vi "Nernst____Newtest.vi"() -> ()   [LabVIEW 2020]
panel:
  out "Temperature Status":i32(ring) items=["TemperatureUnknown"=0, "Stable"=1, "Tracking"=2, "Near"=5, "Chasing"=6, "Filling"=7, "Standby"=10, "Disabled"=13, "ImpedanceNotFunction"=14, "TempFailure"=15]
  out "Field Status":i32(ring) items=["MagnetUnknown"=0, "StablePersistent"=1, "WarmingSwitch"=2, "CoolingSwitch"=3, "StableDriven"=4, "Iterating"=5, "Charging"=6, "Discharging"=7, "CurrentError"=8, "MagnetFailure"=15]
  in  "Field":dbl[](array[numeric])
  out "Temp(A)":dbl
  out "Numeric":dbl
  in  "START":bool
  in  "T cold(A)":dbl
  in  "T hot(B)":dbl
  in  "Remote":bool=TRUE
  in  "IP address":string="10.128.163.210"
  in  "PPMS T(K)":dbl
  in  "Magnetic Field(Oe)":dbl
  in  "Pressure(GPa)":string
  in  "Heater Rate":string="50"
  in  "Heater Output":string="1"
  in  "Heater Mode":string="1"
  in  "Heater range":string="2"
  in  "Starting B":dbl
  in  "starting A":dbl
  out "save file Path":path=path "C:/DATA/Rui/testN1.dat.dat"
  in  "save file input":path=path "C:/DATA/Rui/testN1.dat"
  in  "Voltmeter":string="07"
  in  "T controller":string="12"
  out "Field\nStatus 2":i32(ring) items=["MagnetUnknown"=0, "StablePersistent"=1, "WarmingSwitch"=2, "CoolingSwitch"=3, "StableDriven"=4, "Iterating"=5, "Charging"=6, "Discharging"=7, "CurrentError"=8, "MagnetFailure"=15]
  in  "Cooling/Warming field":dbl[](array[numeric])
  in  "Field (Oe)":dbl[](array[numeric])=[0.0, 0.0, 0.0, 0.0, 0.0, 0.0, 0.0, 0.0]
  in  "Field Rate(Oe/sec)":dbl=100.0
  in  "Wait for T(s)":dbl=50.0
  in  "Wait for Field(s)":dbl=60.0
  in  "Wait For Temperature":bool=TRUE
  in  "T rate(K/min)":dbl=10.0
  in  "Delta T (TA-PPMST)":dbl[](array[numeric])=[0.0]
  in  "PPMST (K)":dbl[](array[numeric])=[0.0, 0.0]
  out "TIming(ms)":dbl
  in  "Time(ms)":dbl[](array[numeric])
  out "T gradient(K)":dbl
  in  "T gradient(K)":dbl[](array[numeric])
  out "Delta V(mV)":dbl
  out "T(A)(K)":dbl
  out "T(B)(K)":dbl
  in  "Tab Control":enum32{"V vs T", "V vs H"}(tab)
  out "XY Graph":cluster{"Y":dbl[], "Y":dbl[]}[](graph)
  out "XY Graph 2":cluster{"Y":dbl[], "Y":dbl[]}[](graph)
  in  "T Hot(A)":dbl[](array[numeric])
  in  "Delt V":dbl[](array[numeric])
  in  "T cold(B)":dbl[](array[numeric])
  # "Heater setups"
  # "GPIB Address"
  # "Save File Path"
  # "Environment setup"
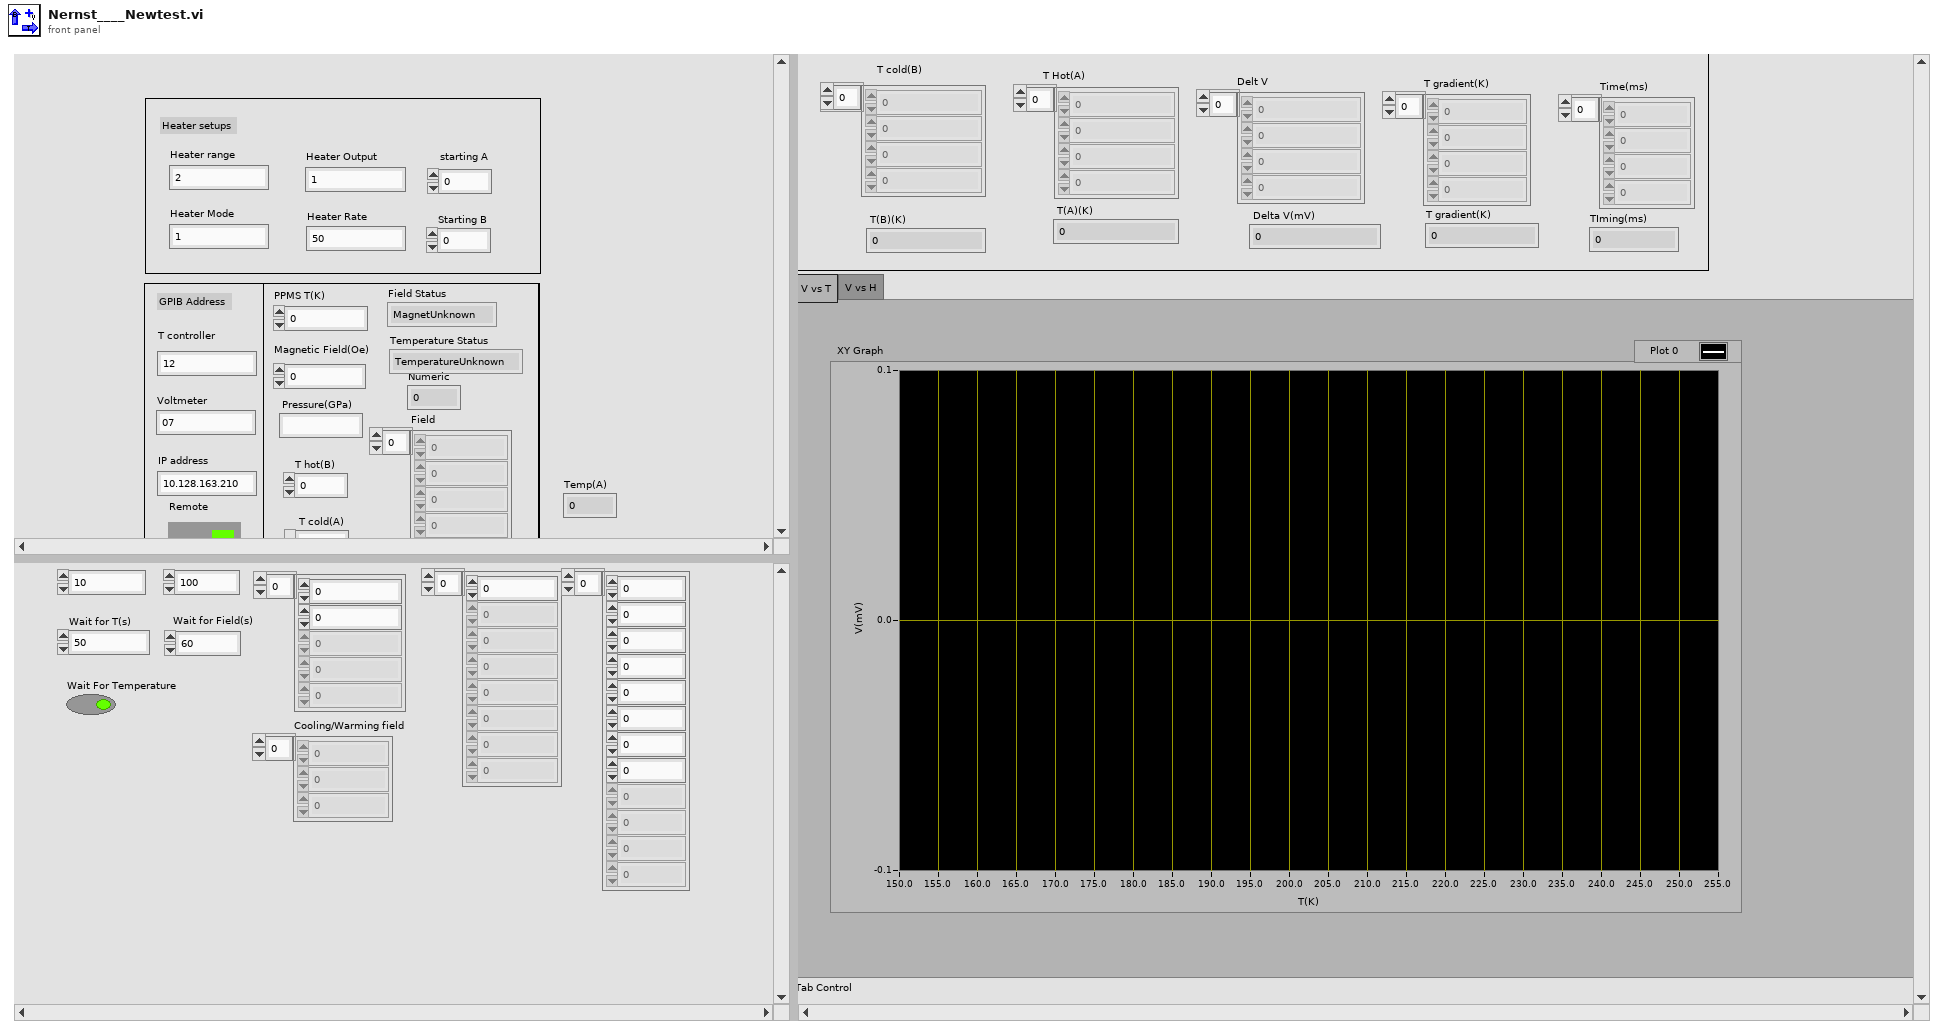
[diagram p1: front panel]
types:
  T1 = enum16{"open", "replace", "create", "open or create", "replace or create", "replace or create with confirmation"}
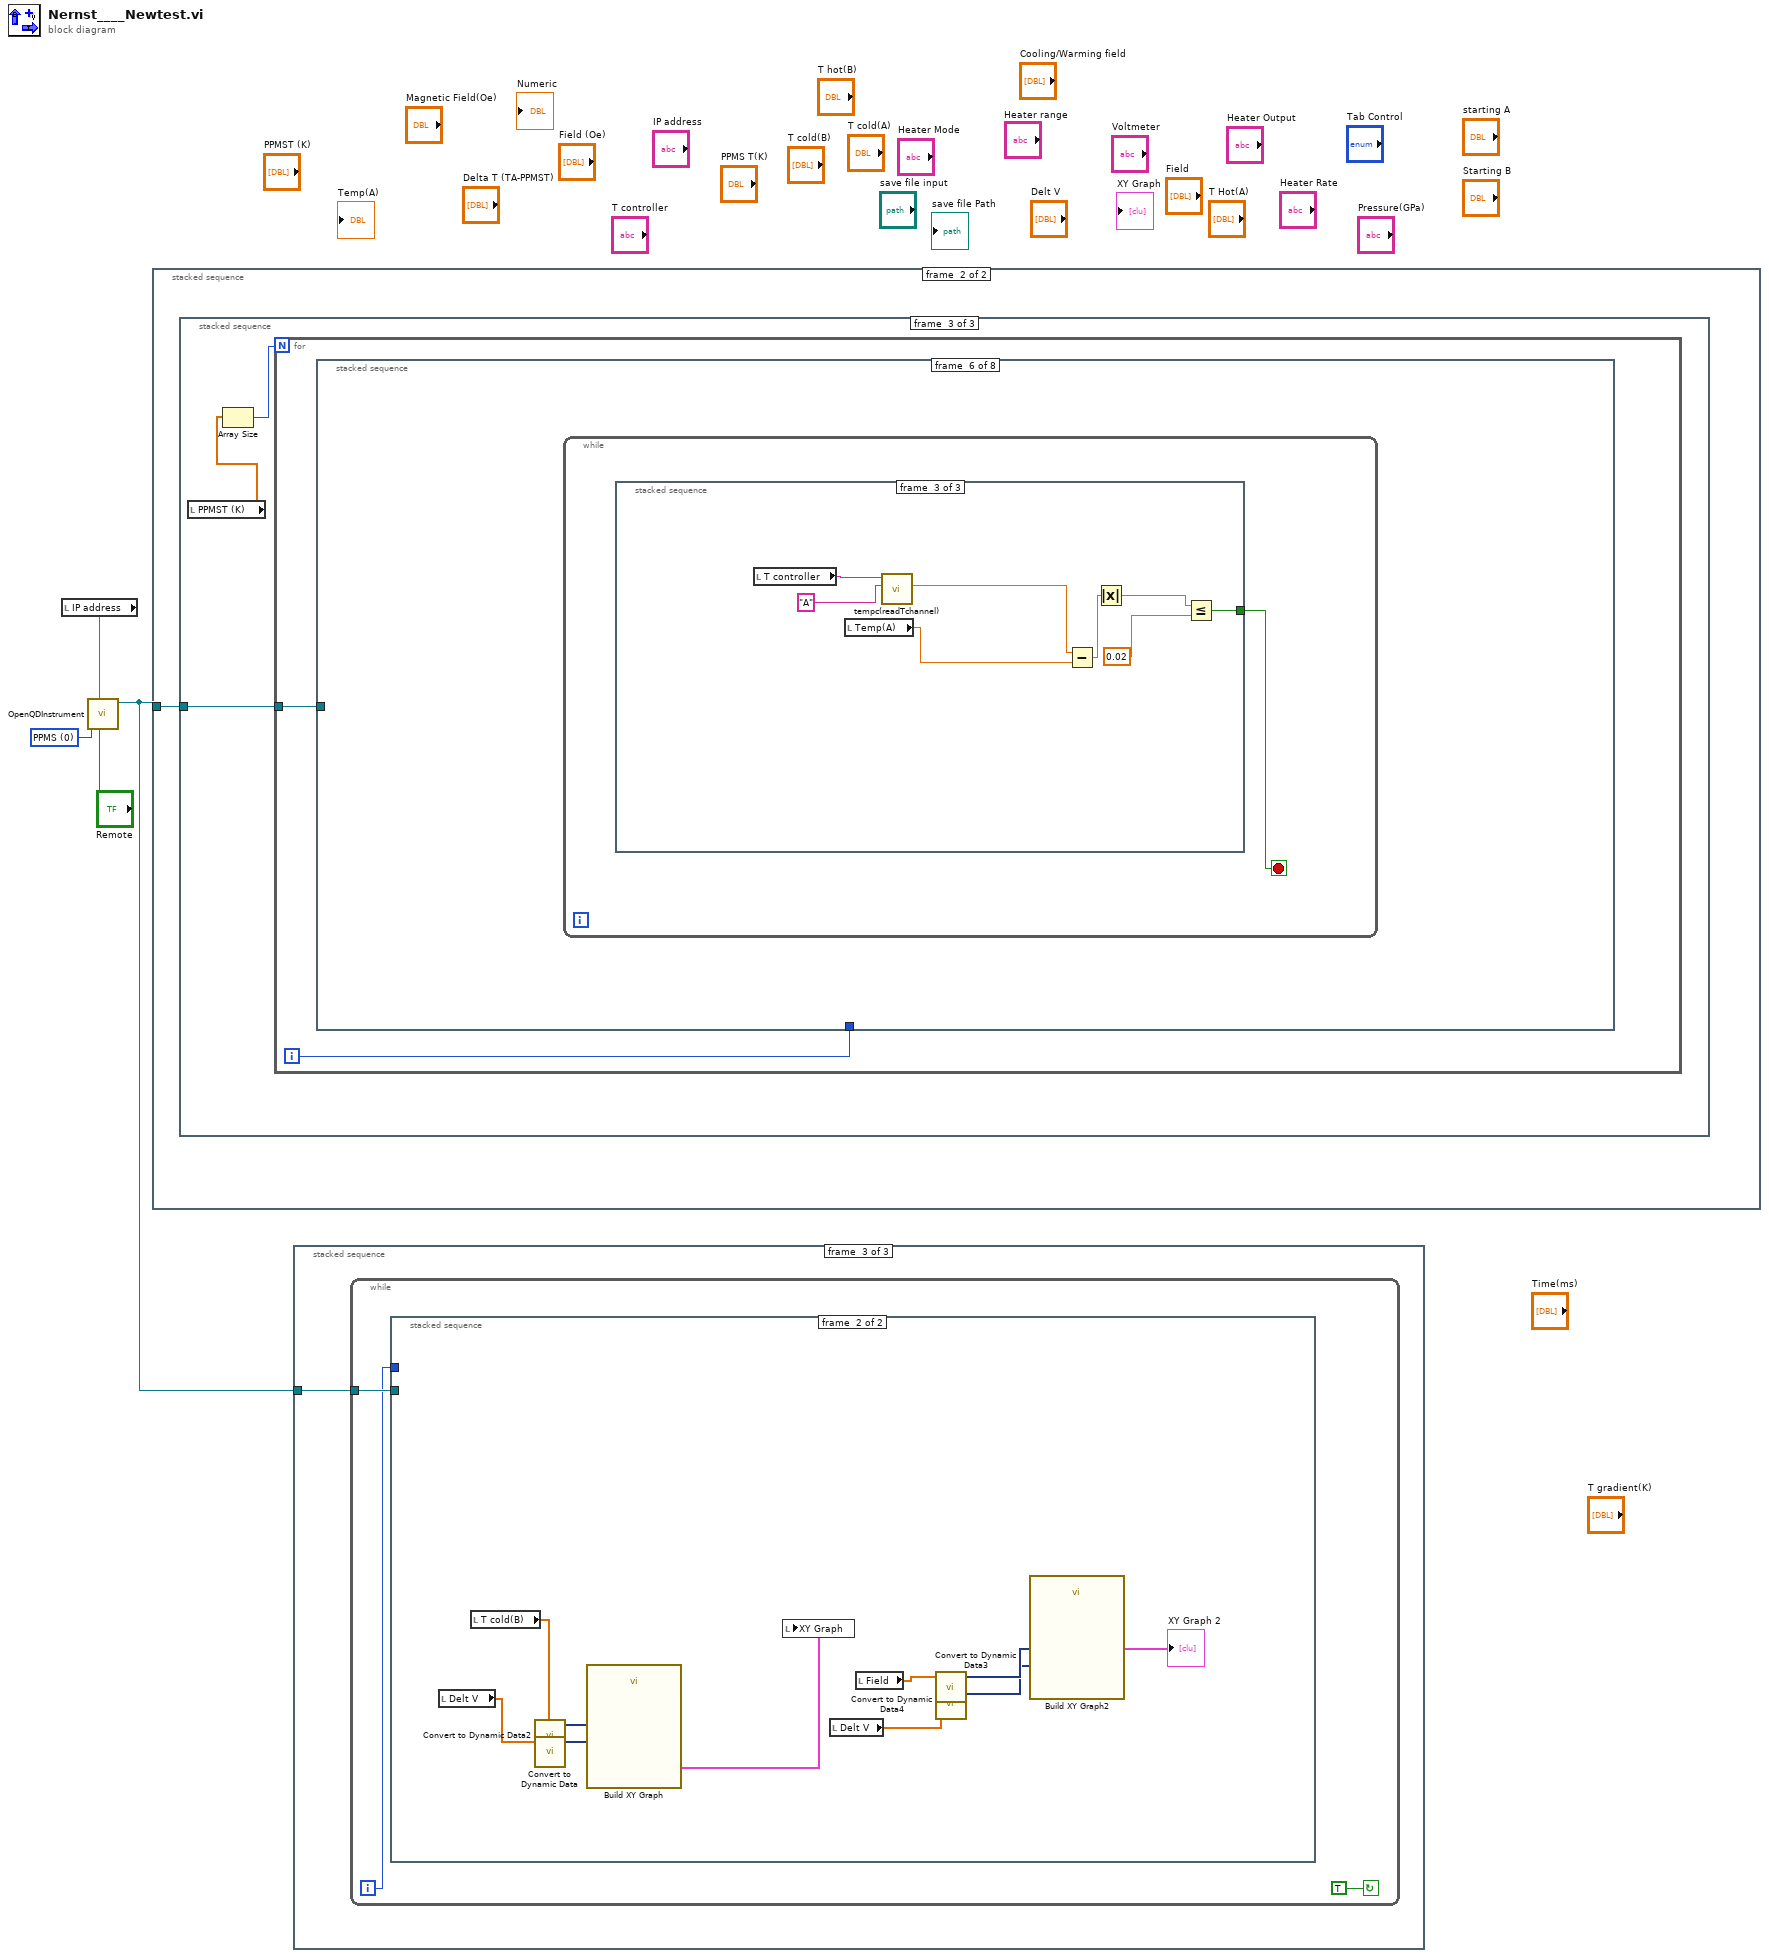
[diagram p0: block diagram]
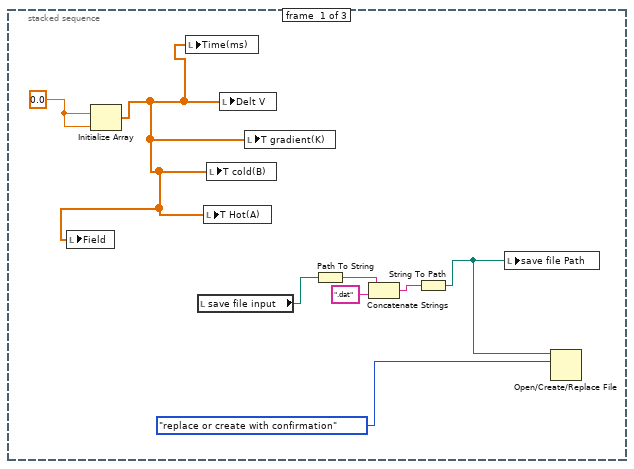
[diagram p2: hidden frame]
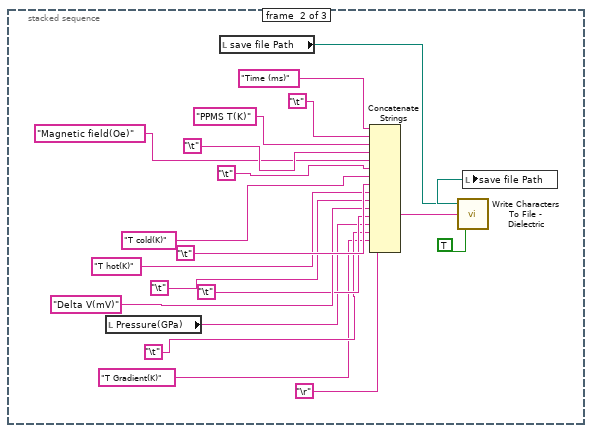
[diagram p3: hidden frame]
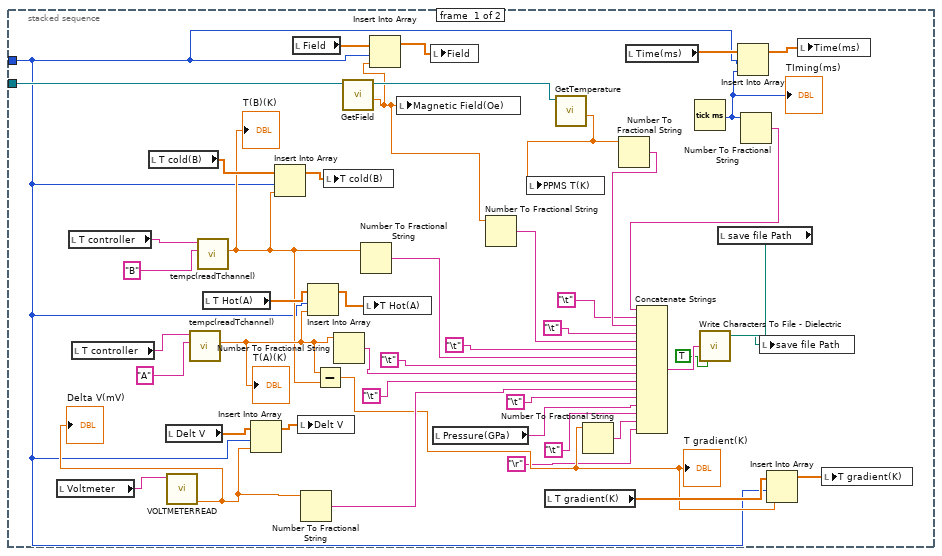
[diagram p4: hidden frame]
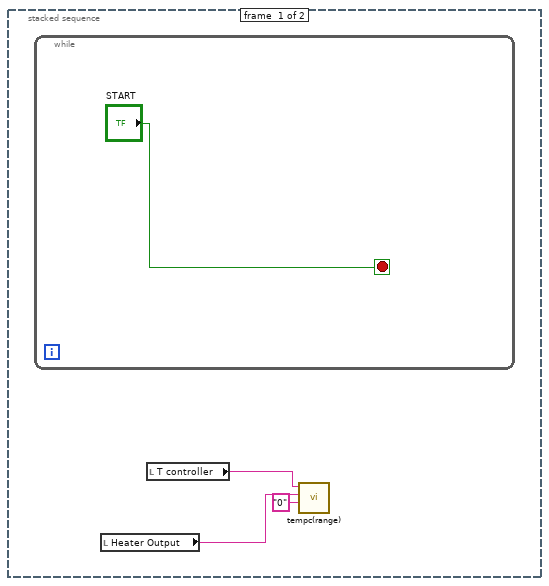
[diagram p5: hidden frame]
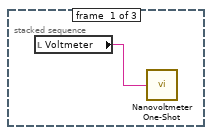
[diagram p6: hidden frame]
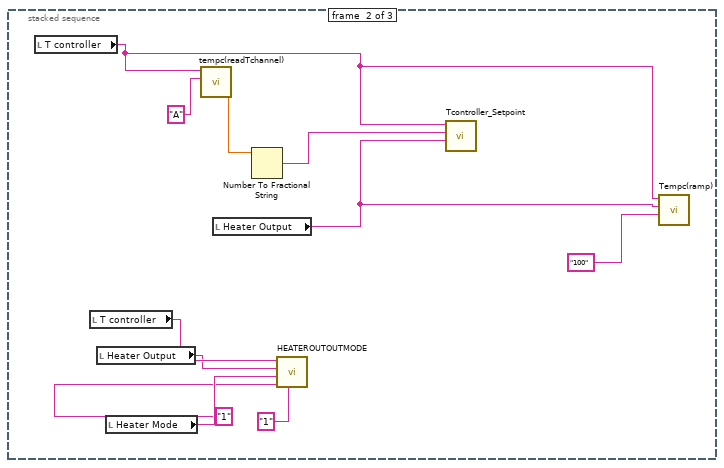
[diagram p7: hidden frame]
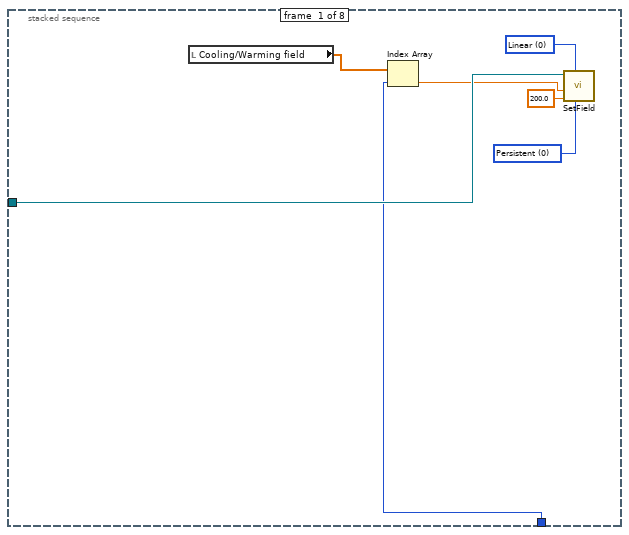
[diagram p8: hidden frame]
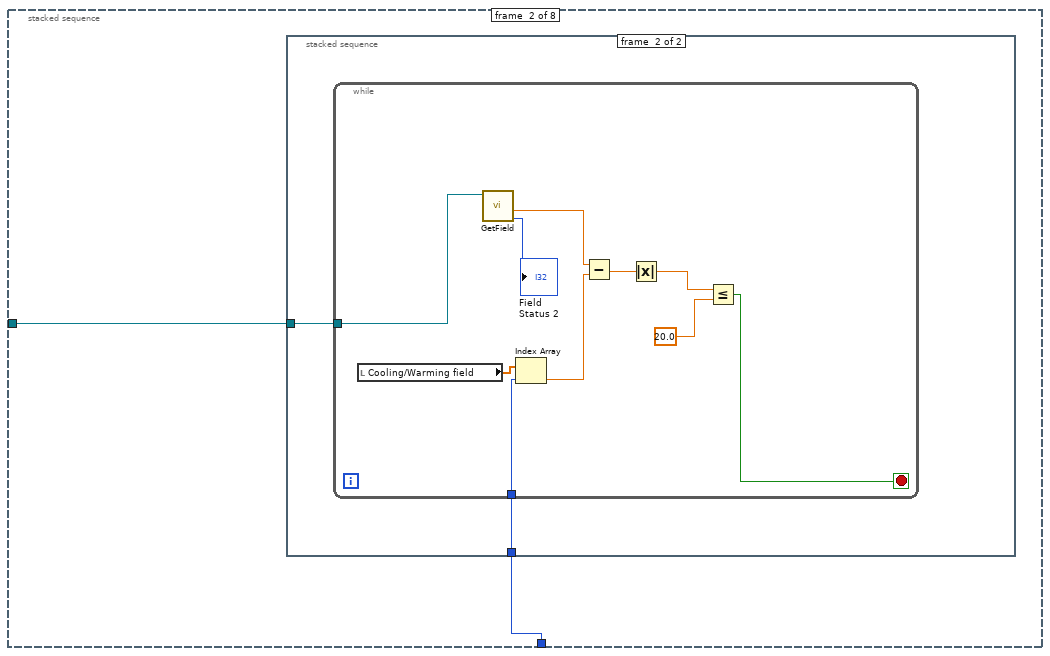
[diagram p9: hidden frame]
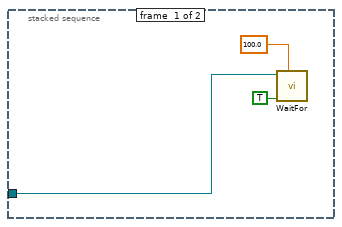
[diagram p10: hidden frame]
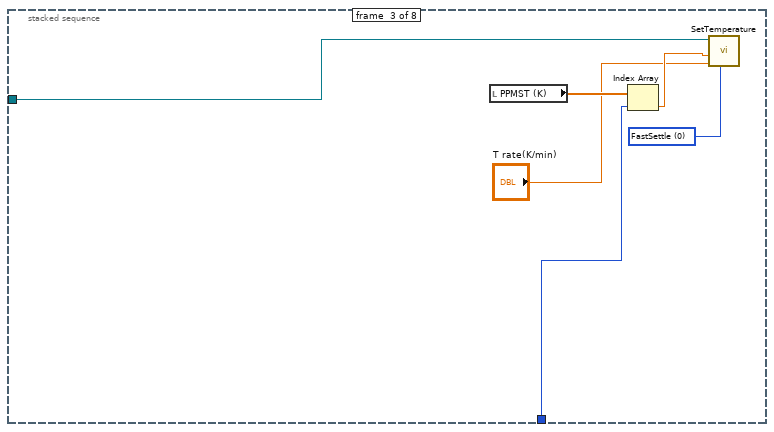
[diagram p11: hidden frame]
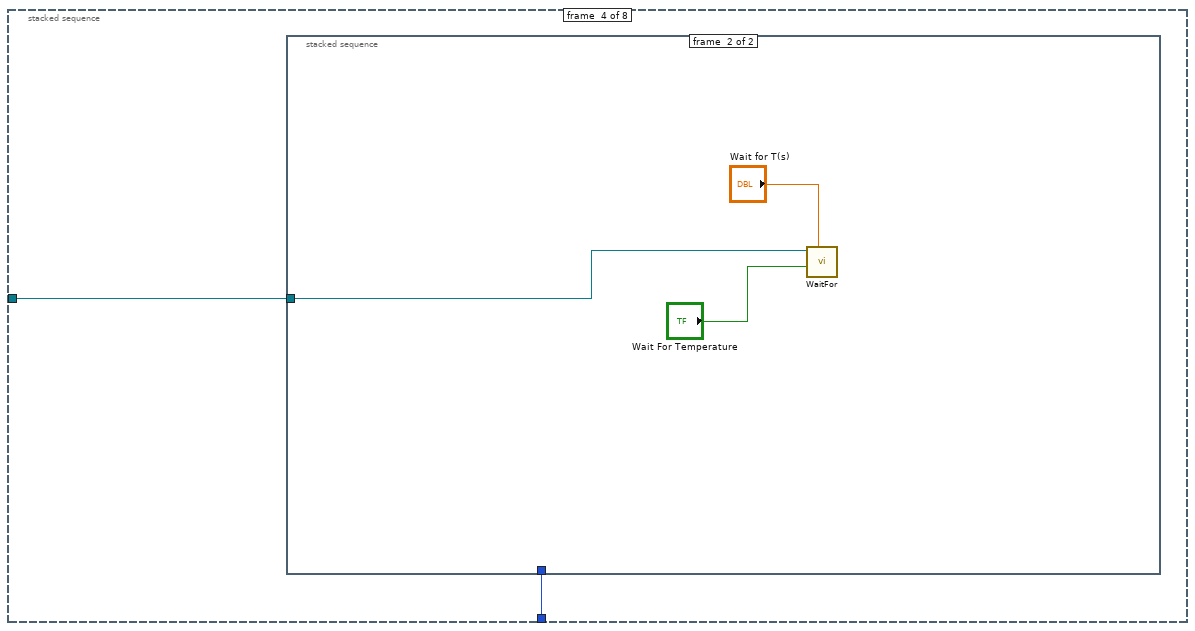
[diagram p12: hidden frame]
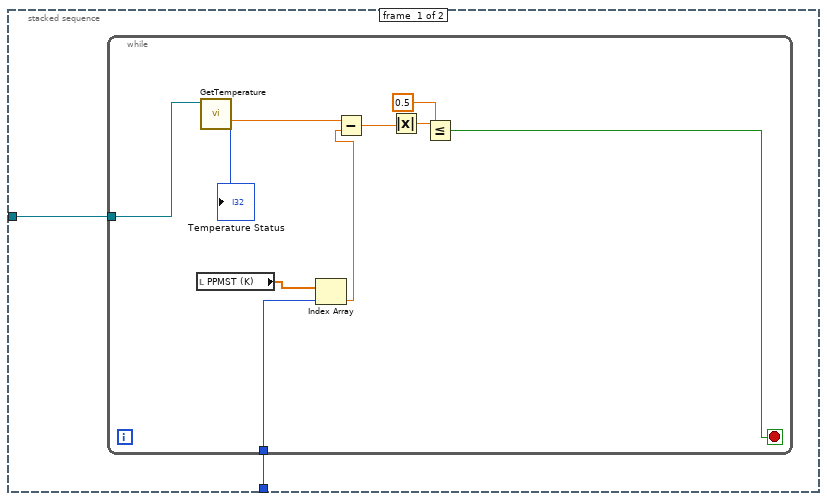
[diagram p13: hidden frame]
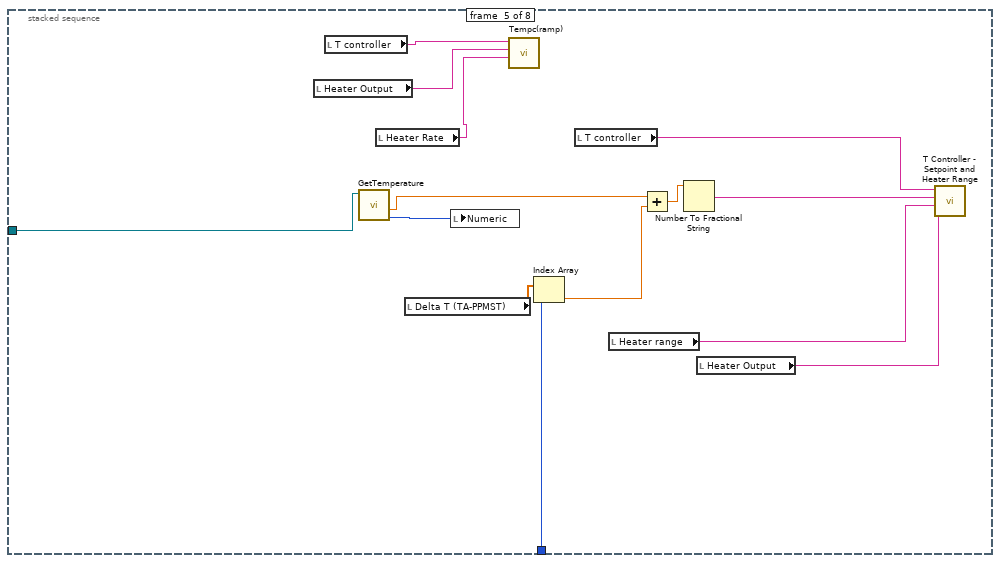
[diagram p14: hidden frame]
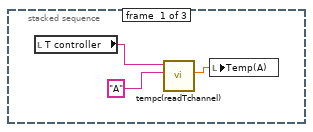
[diagram p15: hidden frame]
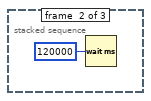
[diagram p16: hidden frame]
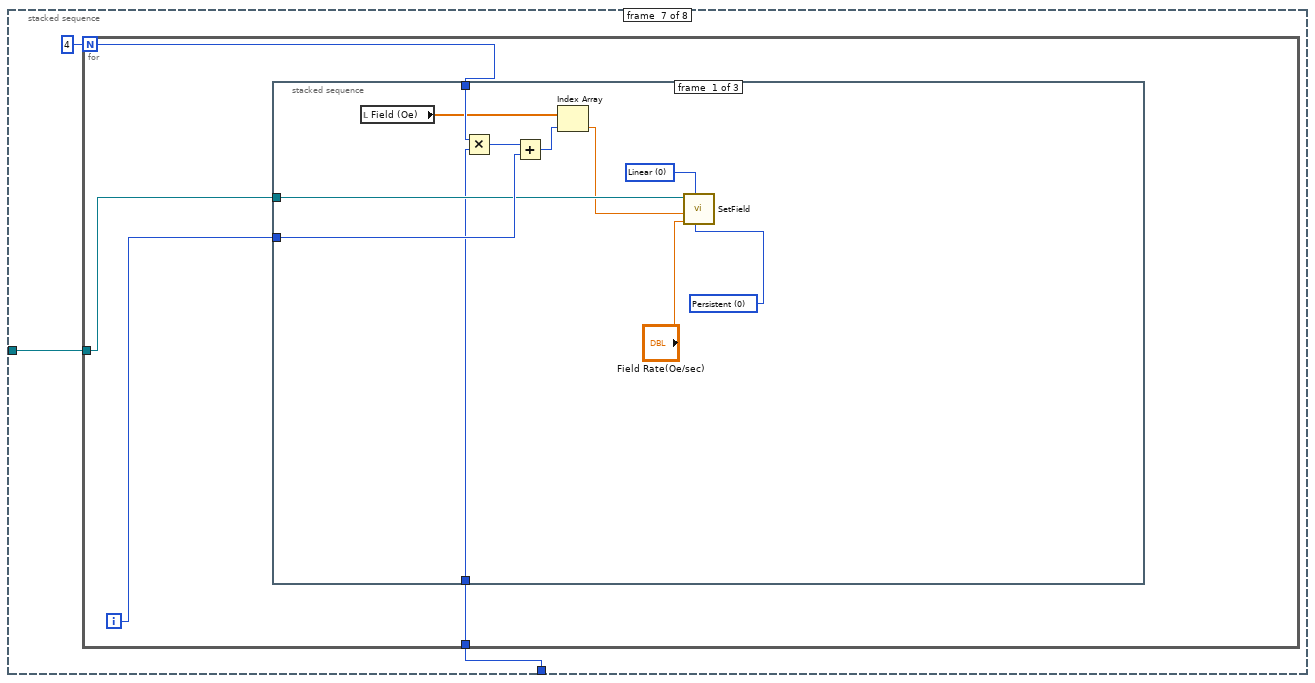
[diagram p17: hidden frame]
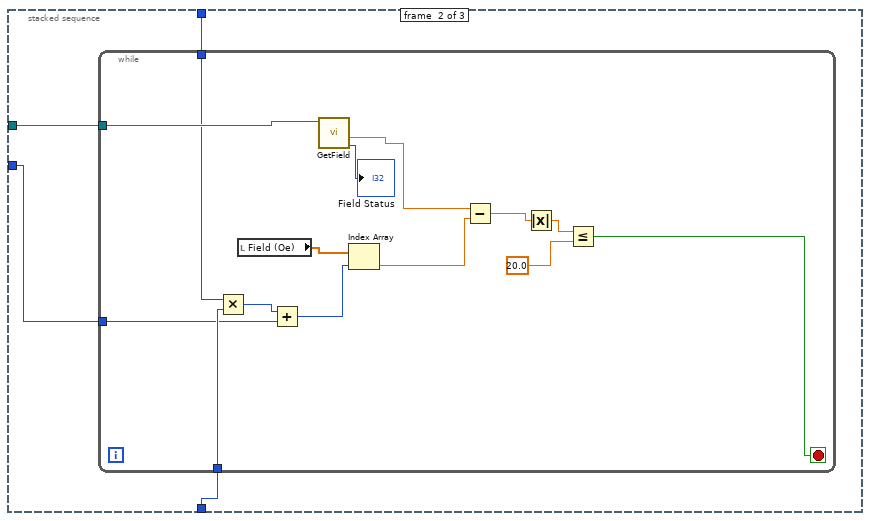
[diagram p18: hidden frame]
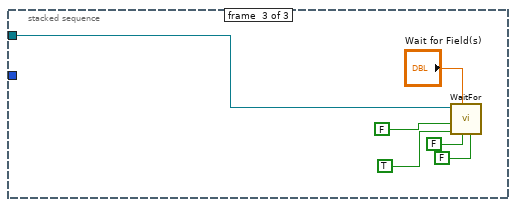
[diagram p19: hidden frame]
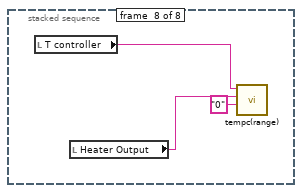
[diagram p20: hidden frame]
diagram:
  w2 = 0 items=["PPMS", "VersaLab", "DynaCool", "SVSM"] ("Instrument Type")
  n1 = local read "IP address"() -> (w4:string)
  n2 = call "OpenQDInstrument.vi"("Remote"="Remote", "IP Address"=w4, "Instrument Type"=w2) -> ("Instrument Ref"=w1:refnum<k24>)  [unwired: 5 in, 1 out]
  n3 = stacked-sequence {
    tunnel: w1 -> [_ w9]
    frame #0 {
      n4 = while {
        stop <- "START" stop-if-true
      }
      n5 = local read "Heater Output"() -> (w6:string)
      n6 = local read "T controller"() -> (w7:string)
      n7 = call "tempc(range).vi"("Heater ramge"="0", "Heater Output"=w6, "GPIB"=w7) -> ()  [unwired: 9 in]
    }
    frame #1 {
      n8 = stacked-sequence {
        tunnel: w9 -> [_ _ w24]
        frame #0 {
          n9 = local read "Voltmeter"() -> (w10:string)
          n10 = call "Nanovoltmeter One-Shot.vi"("GPIB address"=w10) -> ()
        }
        frame #1 {
          n11 = local read "T controller"() -> (w13:string)
          n12 = local read "T controller"() -> (w18:string)
          n13 = local read "Heater Output"() -> (w17:string)
          n14 = local read "Heater Mode"() -> (w16:string)
          n15 = call "tempc(readTchannel).vi"("input"="A", "address string"=w13) -> ("Temp"=w20:dbl)  [unwired: 9 in]
          n16 = local read "Heater Output"() -> (w12:string)
          n17 = Number To Fractional String(number=w20) -> (F-format string=w19:string)  [unwired: 3 in]
          n18 = call "HEATEROUTOUTMODE.vi"("poweruo enable"="1", "Input"="1", "Mode"=w16, "OUtput"=w17, "GPIB"=w18) -> ()  [unwired: 7 in]
          n19 = call "Tcontroller_Setpoint.vi"("OUTPUT"=w12, "SETPOINT"=w19, "GPIB"=w13) -> ()  [unwired: 9 in]
          n20 = call "Tempc(ramp).vi"("Rate Value"="100", "Output"=w12, "DPIB Add"=w13) -> ()  [unwired: 9 in]
        }
        frame #2 {
          n21 = local read "PPMST (K)"() -> (w23:dbl[])
          n22 = Array Size(array=w23) -> (size(s)=w22:i32)
          n23 = for {
            N: w22 -> [_]
            tunnel: w24 -> [w26]
            i -> [w25]
            n24 = stacked-sequence {
              tunnel: w26 -> [w33 w35 w56 w58 w79 _ w103 _]
              tunnel: w25 -> [w31 w34 w51 w57 w74 _ w101 _]
              frame #0 {
                w27 = 0 items=["Persistent", "Driven"] ("Mode")
                w28 = 0 items=["Linear", "NoOvershoot", "Oscillate"] ("Approach")
                n25 = local read "Cooling/Warming field"() -> (w32:dbl[])
                n26 = Index Array(array=w32, index=w31) -> (element=w30:dbl)
                n27 = call "SetField.vi"("Mode"=w27, "Approach"=w28, "Rate"=200.0, "Field"=w30, "Instrument Ref In"=w33) -> ()  [unwired: 2 in, 3 out]
              }
              frame #1 {
                n28 = stacked-sequence {
                  tunnel: w35 -> [w38 w40]
                  tunnel: w34 -> [_ w39]
                  frame #0 {
                    n29 = call "WaitFor.vi"("Delay"=100.0, "Wait For Field"=TRUE, "Instrument Ref In"=w38) -> ()  [unwired: 7 in, 2 out]
                  }
                  frame #1 {
                    n30 = while {
                      tunnel: w40 -> [w50]
                      tunnel: w39 -> [w48]
                      stop <- w41 stop-if-true
                      n31 = local read "Cooling/Warming field"() -> (w49:dbl[])
                      n32 = call "GetField.vi"("Instrument Ref In"=w50) -> ("Field\nStatus"=→"Field\nStatus 2":i32, "Field"=w47:dbl)  [unwired: 4 in, 3 out]
                      n33 = Index Array(array=w49, index=w48) -> (element=w46:dbl)
                      n34 = Subtract(x=w47, y=w46) -> (x-y=w44:dbl)
                      n35 = Absolute Value(x=w44) -> (abs(x)=w43:dbl)
                      n36 = Less Or Equal?(x=w43, y=20.0) -> (x <= y?=w41:bool)
                    }
                  }
                }
              }
              frame #2 {
                w52 = 0 items=["FastSettle", "NoOvershoot"] ("Approach")
                n37 = local read "PPMST (K)"() -> (w55:dbl[])
                n38 = Index Array(array=w55, index=w51) -> (element=w54:dbl)
                n39 = call "SetTemperature.vi"("Approach"=w52, "Rate"="T rate(K/min)", "Temperature"=w54, "Instrument Ref In"=w56) -> ()  [unwired: 3 in, 3 out]
              }
              frame #3 {
                n40 = stacked-sequence {
                  tunnel: w58 -> [w60 w73]
                  tunnel: w57 -> [w59 _]
                  frame #0 {
                    n41 = while {
                      tunnel: w60 -> [w70]
                      tunnel: w59 -> [w67]
                      stop <- w61 stop-if-true
                      n42 = local read "PPMST (K)"() -> (w68:dbl[])
                      n43 = call "GetTemperature.vi"("Instrument Ref In"=w70) -> ("Temperature\nStatus"=→"Temperature Status":i32, "Temperature"=w65:dbl)  [unwired: 4 in, 3 out]
                      n44 = Index Array(array=w68, index=w67) -> (element=w66:dbl)
                      n45 = Subtract(x=w65, y=w66) -> (x-y=w64:dbl)
                      n46 = Absolute Value(x=w64) -> (abs(x)=w63:dbl)
                      n47 = Less Or Equal?(x=w63, y=0.5) -> (x <= y?=w61:bool)
                    }
                  }
                  frame #1 {
                    n48 = call "WaitFor.vi"("Delay"="Wait for T(s)", "Wait For Temperature"="Wait For Temperature", "Instrument Ref In"=w73) -> ()  [unwired: 7 in, 2 out]
                  }
                }
              }
              frame #4 {
                n49 = local read "Heater Output"() -> (w86:string)
                n50 = local read "T controller"() -> (w87:string)
                n51 = call "GetTemperature.vi"("Instrument Ref In"=w79) -> ("Temperature\nStatus"=w77:i32, "Temperature"=w78:dbl)  [unwired: 4 in, 3 out]
                n52 = local read "Heater Rate"() -> (w85:string)
                n53 = local read "Delta T (TA-PPMST)"() -> (w76:dbl[])
                n54 = local write "Numeric"(w77) -> ()
                n55 = call "Tempc(ramp).vi"("Rate Value"=w85, "Output"=w86, "DPIB Add"=w87) -> ()  [unwired: 9 in]
                n56 = Index Array(array=w76, index=w74) -> (element=w75:dbl)
                n57 = local read "T controller"() -> (w83:string)
                n58 = local read "Heater range"() -> (w81:string)
                n59 = Add(x=w78, y=w75) -> (x+y=w84:dbl)
                n60 = Number To Fractional String(number=w84) -> (F-format string=w82:string)  [unwired: 3 in]
                n61 = local read "Heater Output"() -> (w80:string)
                n62 = call "T Controller - Setpoint and Heater Range.vi"("GPIB address"=w83, "Set T"=w82, "heater range"=w81, "Heater output"=w80) -> ()  [unwired: 3 in]
              }
              frame #5 {
                n63 = while {
                  stop <- w88 stop-if-true
                  n64 = stacked-sequence {
                    tunnel: [_ _ w95] -> w88
                    frame #0 {
                      n65 = local read "T controller"() -> (w91:string)
                      n66 = call "tempc(readTchannel).vi"("input"="A", "address string"=w91) -> ("Temp"=w89:dbl)  [unwired: 9 in]
                      n67 = local write "Temp(A)"(w89) -> ()
                    }
                    frame #1 {
                      n68 = Wait (ms)(milliseconds to wait=u32 120000) -> ()  [unwired: 1 out]
                    }
                    frame #2 {
                      n69 = local read "T controller"() -> (w100:string)
                      n70 = local read "Temp(A)"() -> (w93:dbl)
                      n71 = call "tempc(readTchannel).vi"("input"="A", "address string"=w100) -> ("Temp"=w94:dbl)  [unwired: 9 in]
                      n72 = Subtract(x=w94, y=w93) -> (x-y=w98:dbl)
                      n73 = Absolute Value(x=w98) -> (abs(x)=w97:dbl)
                      n74 = Less Or Equal?(x=w97, y=0.02) -> (x <= y?=w95:bool)
                    }
                  }
                }
              }
              frame #6 {
                n75 = for {
                  N: 4 -> [w104]
                  tunnel: w103 -> [w106]
                  tunnel: w101 -> [w105]
                  i -> [w107]
                  n76 = stacked-sequence {
                    tunnel: w107 -> [w118 w119 _]
                    tunnel: w106 -> [w117 w122 w137]
                    tunnel: w105 -> [w116 w120 _]
                    tunnel: w104 -> [w115 w121 _]
                    frame #0 {
                      w113 = 0 items=["Persistent", "Driven"] ("Mode")
                      w112 = 0 items=["Linear", "NoOvershoot", "Oscillate"] ("Approach")
                      n77 = local read "Field (Oe)"() -> (w110:dbl[])
                      n78 = Multiply(x=w115, y=w116) -> (x*y=w111:i32)
                      n79 = Add(x=w111, y=w118) -> (x+y=w109:i32)
                      n80 = Index Array(array=w110, index=w109) -> (element=w108:dbl)
                      n81 = call "SetField.vi"("Mode"=w113, "Approach"=w112, "Rate"="Field Rate(Oe/sec)", "Field"=w108, "Instrument Ref In"=w117) -> ()  [unwired: 2 in, 3 out]
                    }
                    frame #1 {
                      n82 = while {
                        tunnel: w122 -> [w136]
                        tunnel: w121 -> [w133]
                        tunnel: w120 -> [w132]
                        tunnel: w119 -> [w130]
                        stop <- w123 stop-if-true
                        n83 = Multiply(x=w133, y=w132) -> (x*y=w131:i32)
                        n84 = local read "Field (Oe)"() -> (w134:dbl[])
                        n85 = Add(x=w131, y=w130) -> (x+y=w129:i32)
                        n86 = call "GetField.vi"("Instrument Ref In"=w136) -> ("Field\nStatus"=→"Field Status":i32, "Field"=w128:dbl)  [unwired: 4 in, 3 out]
                        n87 = Index Array(array=w134, index=w129) -> (element=w127:dbl)
                        n88 = Subtract(x=w128, y=w127) -> (x-y=w126:dbl)
                        n89 = Absolute Value(x=w126) -> (abs(x)=w125:dbl)
                        n90 = Less Or Equal?(x=w125, y=20.0) -> (x <= y?=w123:bool)
                      }
                    }
                    frame #2 {
                      n91 = call "WaitFor.vi"("Wait For Chamber"=FALSE, "Wait For Position"=FALSE, "Delay"="Wait for Field(s)", "Wait For Field"=TRUE, "Wait For Temperature"=FALSE, "Instrument Ref In"=w137) -> ()  [unwired: 4 in, 2 out]
                    }
                  }
                }
              }
              frame #7 {
                n92 = local read "T controller"() -> (w145:string)
                n93 = local read "Heater Output"() -> (w144:string)
                n94 = call "tempc(range).vi"("Heater ramge"="0", "Heater Output"=w144, "GPIB"=w145) -> ()  [unwired: 9 in]
              }
            }
          }
        }
      }
    }
  }
  n95 = stacked-sequence {
    tunnel: w1 -> [_ _ w174]
    frame #0 {
      w147 = 0.0 ("element")
      n96 = Initialize Array(w147, w147) -> (w146:dbl[])
      n97 = local write "Field"(w146) -> ()
      n98 = local write "Time(ms)"(w146) -> ()
      n99 = local read "save file input"() -> (w150:path)
      n100 = local write "T Hot(A)"(w146) -> ()
      n101 = local write "T cold(B)"(w146) -> ()
      n102 = local write "Delt V"(w146) -> ()
      n103 = local write "T gradient(K)"(w146) -> ()
      n104 = Path To String(path=w150) -> (string=w151:string)
      n105 = Concatenate Strings(w151, ".dat" ("string")) -> (w152:string)
      n106 = String To Path(string=w152) -> (path=w153:path)
      n107 = local write "save file Path"(w153) -> ()
      n108 = Open/Create/Replace File(file path (use dialog)=w153, operation (0:open)=T1."replace or create with confirmation") -> ()  [unwired: 4 in, 3 out]
    }
    frame #1 {
      n109 = local read "Pressure(GPa)"() -> (w157:string)
      n110 = local read "save file Path"() -> (w171:path)
      n111 = Concatenate Strings("Time (ms)" ("string"), "\t", "PPMS T(K)" ("string"), "\t", "Magnetic field(Oe)" ("string"), "\t", "T cold(K)" ("string"), "\t", "T hot(K)" ("string"), "\t", "Delta V(mV)" ("string"), "\t", w157, "\t", "T Gradient(K)" ("string"), "\r") -> (w173:string)
      n112 = call "Write Characters To File - Dielectric.vi"("append to file? (new file:F)"=TRUE, "character string"=w173, "file path (dialog if empty)"=w171) -> ("new file path (Not A Path if cancelled)"=w172:path)  [unwired: 2 in]
      n113 = local write "save file Path"(w172) -> ()
    }
    frame #2 {
      n114 = while {
        tunnel: w174 -> [w177]
        i -> [w176]
        stop <- TRUE continue-if-true
        n115 = stacked-sequence {
          tunnel: w177 -> [w197 _]
          tunnel: w176 -> [w179 _]
          frame #0 {
            n116 = local read "Voltmeter"() -> (w208:string)
            n117 = local read "T controller"() -> (w206:string)
            n118 = local read "T controller"() -> (w207:string)
            n119 = local read "T cold(B)"() -> (w209:dbl[])
            n120 = local read "Delt V"() -> (w213:dbl[])
            n121 = call "VOLTMETERREAD.vi"("String"=w208) -> ("number 2"=w193:dbl)  [unwired: 10 in]
            "Delta V(mV)" <- w193
            n122 = call "tempc(readTchannel).vi"("input"="A", "address string"=w207) -> ("Temp"=w189:dbl)  [unwired: 9 in]
            "T(A)(K)" <- w189
            n123 = call "tempc(readTchannel).vi"("input"="B", "address string"=w206) -> ("Temp"=w188:dbl)  [unwired: 9 in]
            "T(B)(K)" <- w188
            n124 = local read "T Hot(A)"() -> (w211:dbl[])
            n125 = Insert Into Array(array=w213, index=w179, new element=w193) -> (w214:dbl[])
            n126 = Insert Into Array(array=w209, index=w179, new element=w188) -> (w210:dbl[])
            n127 = local read "Field"() -> (w196:dbl[])
            n128 = local write "Delt V"(w214) -> ()
            n129 = Number To Fractional String(number=w193) -> (F-format string=w215:string)  [unwired: 3 in]
            n130 = Insert Into Array(array=w211, index=w179, new element=w189) -> (w212:dbl[])
            n131 = Subtract(x=w189, y=w188) -> (x-y=w185:dbl)
            "T gradient(K)" <- w185
            n132 = local write "T cold(B)"(w210) -> ()
            n133 = Number To Fractional String(number=w189) -> (F-format string=w216:string)  [unwired: 3 in]
            n134 = call "GetField.vi"("Instrument Ref In"=w197) -> ("Field"=w195:dbl, "Instrument Ref Out"=w223:refnum<k24>)  [unwired: 4 in, 3 out]
            n135 = Number To Fractional String(number=w188) -> (F-format string=w217:string)  [unwired: 3 in]
            n136 = local write "T Hot(A)"(w212) -> ()
            n137 = Insert Into Array(array=w196, index=w179, new element=w195) -> (w194:dbl[])
            n138 = local write "Magnetic Field(Oe)"(w195) -> ()
            n139 = local write "Field"(w194) -> ()
            n140 = local read "Pressure(GPa)"() -> (w221:string)
            n141 = Number To Fractional String(number=w195) -> (F-format string=w222:string)  [unwired: 3 in]
            n142 = local read "T gradient(K)"() -> (w187:dbl[])
            n143 = call "GetTemperature.vi"("Instrument Ref In"=w223) -> ("Temperature"=w224:dbl)  [unwired: 4 in, 4 out]
            n144 = local write "PPMS T(K)"(w224) -> ()
            n145 = Number To Fractional String(number=w185) -> (F-format string=w184:string)  [unwired: 3 in]
            n146 = Number To Fractional String(number=w224) -> (F-format string=w192:string)  [unwired: 3 in]
            n147 = local read "Time(ms)"() -> (w181:dbl[])
            n148 = Tick Count (ms)() -> (millisecond timer value=w178:u32)
            "TIming(ms)" <- w178
            n149 = local read "save file Path"() -> (w220:path)
            n150 = Insert Into Array(array=w181, index=w179, new element=w178) -> (w180:dbl[])
            n151 = Number To Fractional String(number=w178) -> (F-format string=w191:string)  [unwired: 3 in]
            n152 = Concatenate Strings(w191, "\t", w192, "\t", w222, "\t", w217, "\t", w216, "\t", w215, "\t", w221, "\t", w184, "\r") -> (w218:string)
            n153 = call "Write Characters To File - Dielectric.vi"("append to file? (new file:F)"=TRUE, "character string"=w218, "file path (dialog if empty)"=w220) -> ("new file path (Not A Path if cancelled)"=w219:path)  [unwired: 2 in]
            n154 = local write "save file Path"(w219) -> ()
            n155 = Insert Into Array(array=w187, index=w179, new element=w185) -> (w186:dbl[])
            n156 = local write "Time(ms)"(w180) -> ()
            n157 = local write "T gradient(K)"(w186) -> ()
          }
          frame #1 {
            n158 = local read "Delt V"() -> (w233:dbl[])
            n159 = local read "T cold(B)"() -> (w231:dbl[])
            n160 = call "Convert to Dynamic Data2"("Array"=w231) -> ("Dynamic Data Type"=w230:dynamicdata)  [unwired: 3 in]
            n161 = call "Convert to Dynamic Data"("Array"=w233) -> ("Dynamic Data Type"=w232:dynamicdata)  [unwired: 3 in]
            n162 = call "Build XY Graph"("Y Input"=w232, "X Input"=w230) -> ("XY Graph"=w234:cluster{"X":dbl[], "Y":dbl[]}[])  [unwired: 8 in, 1 out]
            n163 = local write "XY Graph"(w234) -> ()
            n164 = local read "Delt V"() -> (w226:dbl[])
            n165 = local read "Field"() -> (w228:dbl[])
            n166 = call "Convert to Dynamic Data3"("Array"=w228) -> ("Dynamic Data Type"=w227:dynamicdata)  [unwired: 3 in]
            n167 = call "Convert to Dynamic Data4"("Array"=w226) -> ("Dynamic Data Type"=w225:dynamicdata)  [unwired: 3 in]
            n168 = call "Build XY Graph2"("Y Input"=w225, "X Input"=w227) -> ("XY Graph"=→"XY Graph 2":cluster{"X":dbl[], "Y":dbl[]}[])  [unwired: 8 in, 1 out]
          }
        }
      }
    }
  }
